vi "Power Output Append Group Data Fields.vi"(10 "Power Output Results":T1={"Measurement Cycles"=0, "Measurement Data"=[], "Pass?"=FALSE, "Instruments to Use"={"PIM Instrument Record"={"ixInstrument"=0, "sxInstrumentId"="", "sDriverId"="", "sDriverType"="", "sSerialNumber"="", "tLastCalibration"=timestamp(0 s since 1904-01-01), "tCalibrationDue"=timestamp(0 s since 1904-01-01), "sConfiguration"=""}, "PWM Instrument Record"={"ixInstrument"=0, "sxInstrumentId"="", "sDriverId"="", "sDriverType"="", "sSerialNumber"="", "tLastCalibration"=timestamp(0 s since 1904-01-01), "tCalibrationDue"=timestamp(0 s since 1904-01-01), "sConfiguration"=""}}, "Power Output Test Parameters"={"Stimulus"={"Frequency Type"=enum."Band Edges", "Frequency Ranges"=[], "TX 1 Frequency (MHz)"={"Min"=0.0, "Max"=0.0}, "TX 2 Frequency (MHz)"={"Min"=0.0, "Max"=0.0}, "RX Frequency (MHz)"={"Min"=0.0, "Max"=0.0}, "Pad Model Number"="", "Pad Serial Number"="", "Pad Values"=[]}, "Measurement"={"DUT Port"=enum."Port 1", "Direction"=0, "Frequency Step Size"=0}, "Display"={"Frequency"={"Min"=-1.0, "Max"=-1.0}, "Power"={"Min"=-1, "Max"=-1}}, "Limit"={"Min Power (dBm)"=44.0}, "Calibration"={"Calibrated?"=FALSE}}, "Calculated Values"={"C1 PWM Power Min (dBm)"=0.0, "C1 PWM Power Max (dBm)"=0.0, "C1 PIM Power Min (dBm)"=0.0, "C1 PIM Power Max (dBm)"=0.0, "C2 PWM Power Min (dBm)"=0.0, "C2 PWM Power Max (dBm)"=0.0, "C2 PIM Power Min (dBm)"=0.0, "C2 PIM Power Max (dBm)"=0.0}} {"Power Output Test Parameters"."Measurement"."Frequency Step Size" items=["0.2", "0.4", "1.0", "2.0", "4.0"]; "Power Output Test Parameters"."Measurement"."Direction" items=["Reverse", "Forward", "Auxiliary"]}, 11 "Fields In":T14[](array[typedef])) -> (3 "Fields Out":T14[](array[typedef]))   [LabVIEW 2011]
uses:
  server/database/Fields/Field Record.ctl
  server/database/Fields/Field DataTypes.ctl
  server/database/Fields/Field NextItem.ctl
  TypeDefs/Power Output Results.ctl
  TypeDefs/Power Output Measurement Data.ctl
  server/database/Stations/Instruments/Instrument Record.ctl
  TypeDefs/Power Output Test Parameters.ctl
  TypeDefs/Power Output Stimulus Parameters.ctl
  TypeDefs/Power Output Measurement Parameters.ctl
  SI.LIB/PIM.LIB/HW IO/DUTport.ctl
  SI.LIB/PIM.LIB/HW IO/MeasMode.ctl
  SI.LIB/PIM.LIB/HW IO/PIM Sweep Step Size.ctl
  TypeDefs/Power Output Display Parameters.ctl
  TypeDefs/Power Output Limit Parameters.ctl
  TypeDefs/Power Output Calibration State.ctl
  TypeDefs/Power Output Calculated Values.ctl
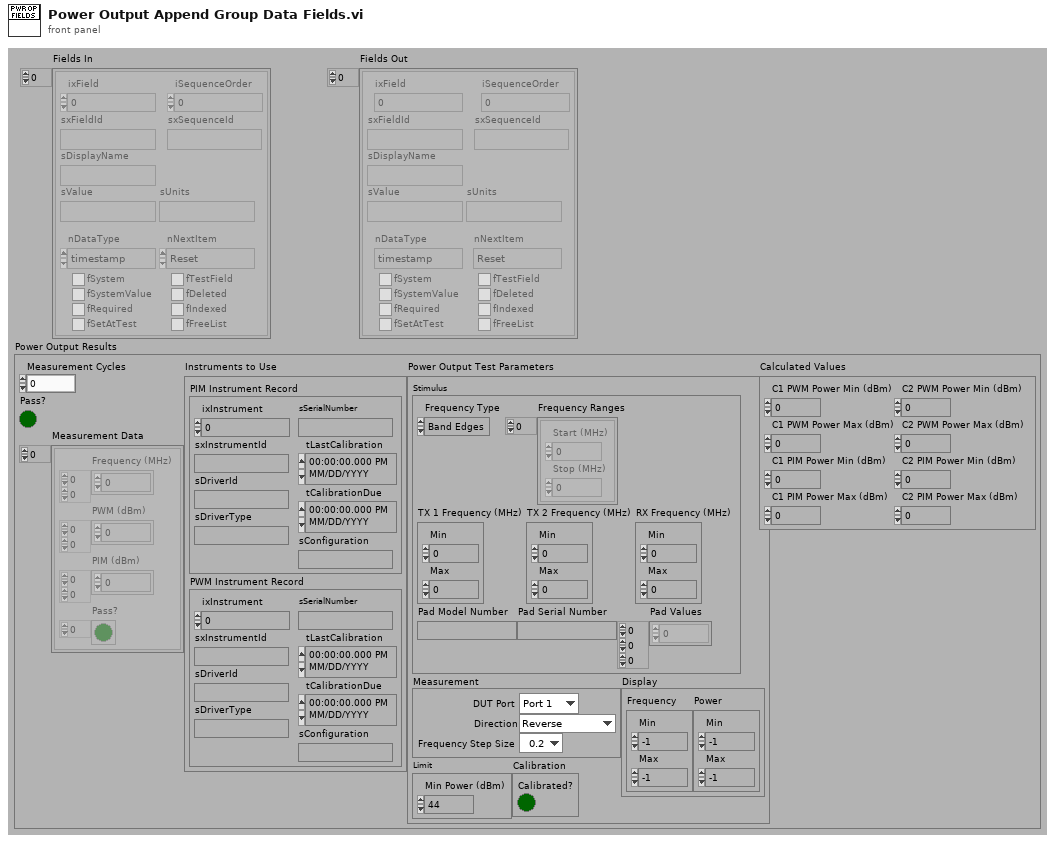
[diagram p1: front panel]
types:
  T1 = typedef "Power Output Results.ctl" = cluster{"Measurement Cycles":i32, "Measurement Data":T2[], "Pass?":bool, "Instruments to Use":cluster{"PIM Instrument Record":T3, "PWM Instrument Record":T3}, "Power Output Test Parameters":T4, "Calculated Values":T13}
  T2 = typedef "Power Output Measurement Data.ctl" = cluster{"Frequency (MHz)":dbl[][], "PWM (dBm)":dbl[][], "PIM (dBm)":dbl[][], "Pass?":bool[]}
  T3 = typedef "Instrument Record.ctl" = cluster{"ixInstrument":i32, "sxInstrumentId":string, "sDriverId":string, "sDriverType":string, "sSerialNumber":string, "tLastCalibration":timestamp, "tCalibrationDue":timestamp, "sConfiguration":string}
  T4 = typedef "Power Output Test Parameters.ctl" = cluster{"Stimulus":T5, "Measurement":T6, "Display":T10, "Limit":T11, "Calibration":T12}
  T5 = typedef "Power Output Stimulus Parameters.ctl" = cluster{"Frequency Type":enum16{"Band Edges", "Custom"}, "Frequency Ranges":cluster{"Start (MHz)":dbl, "Stop (MHz)":dbl}[], "TX 1 Frequency (MHz)":cluster{"Min":dbl, "Max":dbl}, "TX 2 Frequency (MHz)":cluster{"Min":dbl, "Max":dbl}, "RX Frequency (MHz)":cluster{"Min":dbl, "Max":dbl}, "Pad Model Number":string, "Pad Serial Number":string, "Pad Values":dbl[][][]}
  T6 = typedef "Power Output Measurement Parameters.ctl" = cluster{"DUT Port":T7, "Direction":T8, "Frequency Step Size":T9}
  T7 = typedef "DUTport.ctl" = enum16{"Port 1", "Port 2"}
  T8 = typedef "MeasMode.ctl" = u16
  T9 = typedef "PIM Sweep Step Size.ctl" = u16
  T10 = typedef "Power Output Display Parameters.ctl" = cluster{"Frequency":cluster{"Min":dbl, "Max":dbl}, "Power":cluster{"Min":i32, "Max":i32}}
  T11 = typedef "Power Output Limit Parameters.ctl" = cluster{"Min Power (dBm)":dbl}
  T12 = typedef "Power Output Calibration State.ctl" = cluster{"Calibrated?":bool}
  T13 = typedef "Power Output Calculated Values.ctl" = cluster{"C1 PWM Power Min (dBm)":dbl, "C1 PWM Power Max (dBm)":dbl, "C1 PIM Power Min (dBm)":dbl, "C1 PIM Power Max (dBm)":dbl, "C2 PWM Power Min (dBm)":dbl, "C2 PWM Power Max (dBm)":dbl, "C2 PIM Power Min (dBm)":dbl, "C2 PIM Power Max (dBm)":dbl}
  T14 = typedef "Field Record.ctl" = cluster{"ixField":i32, "iSequenceOrder":i32, "sxFieldId":string, "sxSequenceId":string, "sDisplayName":string, "sValue":string, "sUnits":string, "nDataType":T15, "nNextItem":T16, "fSystem":bool, "fSystemValue":bool, "fRequired":bool, "fSetAtTest":bool, "fTestField":bool, "fDeleted":bool, "fIndexed":bool, "fFreeList":bool}
  T15 = typedef "Field DataTypes.ctl" = enum32{"text", "numeric", "list", "timestamp", "boolean"}
  T16 = typedef "Field NextItem.ctl" = enum32{"Reset", "Retain", "Auto-Increment"}
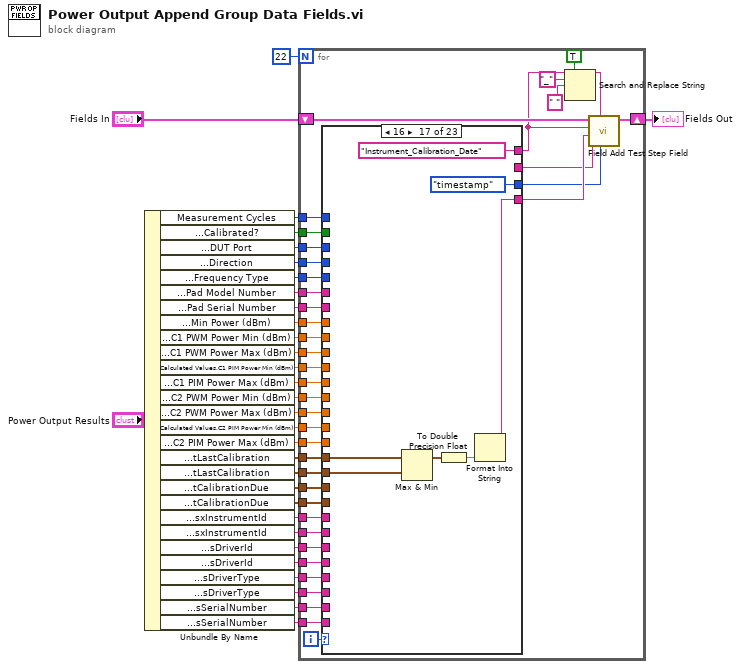
[diagram p0: block diagram]
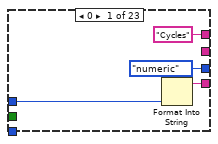
[diagram p2: hidden frame]
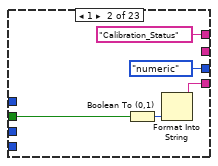
[diagram p3: hidden frame]
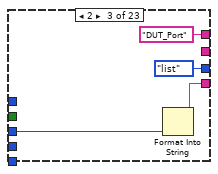
[diagram p4: hidden frame]
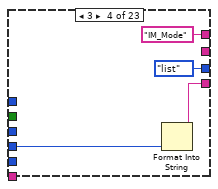
[diagram p5: hidden frame]
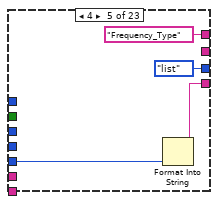
[diagram p6: hidden frame]
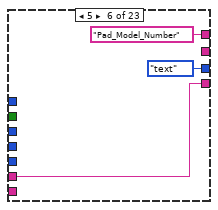
[diagram p7: hidden frame]
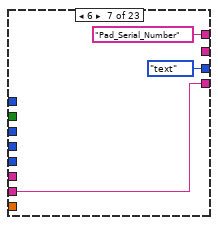
[diagram p8: hidden frame]
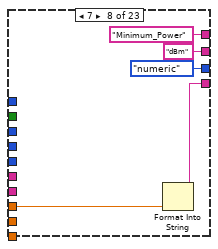
[diagram p9: hidden frame]
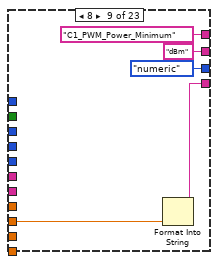
[diagram p10: hidden frame]
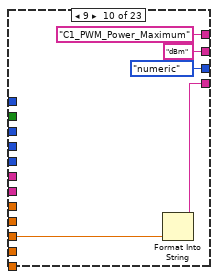
[diagram p11: hidden frame]
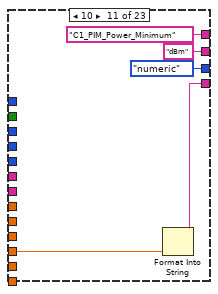
[diagram p12: hidden frame]
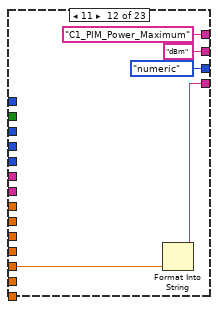
[diagram p13: hidden frame]
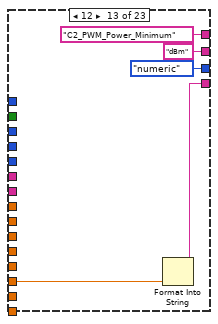
[diagram p14: hidden frame]
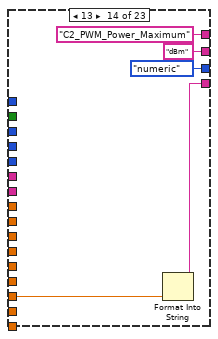
[diagram p15: hidden frame]
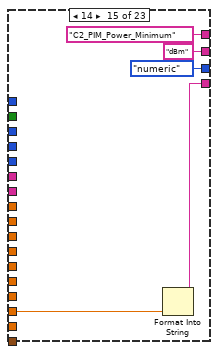
[diagram p16: hidden frame]
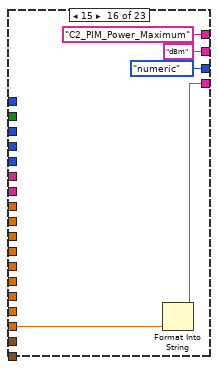
[diagram p17: hidden frame]
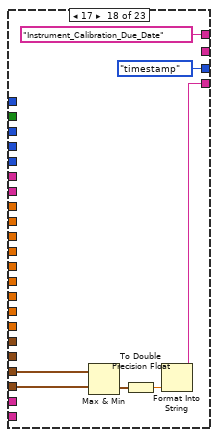
[diagram p18: hidden frame]
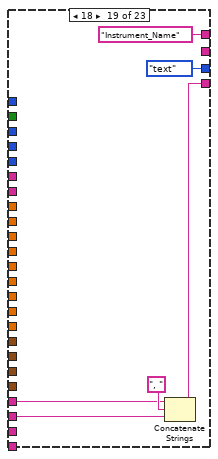
[diagram p19: hidden frame]
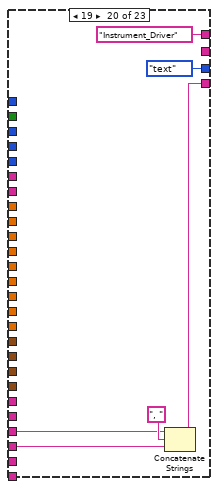
[diagram p20: hidden frame]
diagram:
  n1 = Unbundle By Name("Power Output Results") -> ("Measurement Cycles"=w28:i32, "Power Output Test Parameters.Calibration.Calibrated?"=w27:bool, "Power Output Test Parameters.Measurement.DUT Port"=w26:T7, "Power Output Test Parameters.Measurement.Direction"=w18:T8, "Power Output Test Parameters.Stimulus.Frequency Type"=w19:enum16{"Band Edges", "Custom"}, "Power Output Test Parameters.Stimulus.Pad Model Number"=w11:string, "Power Output Test Parameters.Stimulus.Pad Serial Number"=w10:string, "Power Output Test Parameters.Limit.Min Power (dBm)"=w9:dbl, "Calculated Values.C1 PWM Power Min (dBm)"=w8:dbl, "Calculated Values.C1 PWM Power Max (dBm)"=w7:dbl, "Calculated Values.C1 PIM Power Min (dBm)"=w6:dbl, "Calculated Values.C1 PIM Power Max (dBm)"=w5:dbl, "Calculated Values.C2 PWM Power Min (dBm)"=w4:dbl, "Calculated Values.C2 PWM Power Max (dBm)"=w3:dbl, "Calculated Values.C2 PIM Power Min (dBm)"=w2:dbl, "Calculated Values.C2 PIM Power Max (dBm)"=w1:dbl, "Instruments to Use.PIM Instrument Record.tLastCalibration"=w25:timestamp, "Instruments to Use.PWM Instrument Record.tLastCalibration"=w12:timestamp, "Instruments to Use.PIM Instrument Record.tCalibrationDue"=w24:timestamp, "Instruments to Use.PWM Instrument Record.tCalibrationDue"=w13:timestamp, "Instruments to Use.PIM Instrument Record.sxInstrumentId"=w23:string, "Instruments to Use.PWM Instrument Record.sxInstrumentId"=w17:string, "Instruments to Use.PIM Instrument Record.sDriverId"=w22:string, "Instruments to Use.PWM Instrument Record.sDriverId"=w16:string, "Instruments to Use.PIM Instrument Record.sDriverType"=w21:string, "Instruments to Use.PWM Instrument Record.sDriverType"=w15:string, "Instruments to Use.PIM Instrument Record.sSerialNumber"=w20:string, "Instruments to Use.PWM Instrument Record.sSerialNumber"=w14:string)
  n2 = for {
    N: 22 -> [_]
    shift-right: [w69] -> w31
    shift-left: "Fields In" -> [w70]
    tunnel: w28 -> [w65]
    tunnel: w27 -> [w64]
    tunnel: w26 -> [w63]
    tunnel: w25 -> [w62]
    tunnel: w24 -> [w61]
    tunnel: w23 -> [w60]
    tunnel: w22 -> [w59]
    tunnel: w21 -> [w58]
    tunnel: w20 -> [w57]
    tunnel: w19 -> [w56]
    tunnel: w18 -> [w50]
    tunnel: w17 -> [w49]
    tunnel: w16 -> [w48]
    tunnel: w15 -> [w47]
    tunnel: w14 -> [w46]
    tunnel: w13 -> [w45]
    tunnel: w12 -> [w44]
    tunnel: w11 -> [w43]
    tunnel: w10 -> [w42]
    tunnel: w9 -> [w41]
    tunnel: w8 -> [w40]
    tunnel: w7 -> [w39]
    tunnel: w6 -> [w38]
    tunnel: w5 -> [w37]
    tunnel: w4 -> [w36]
    tunnel: w3 -> [w35]
    tunnel: w2 -> [w34]
    tunnel: w1 -> [w33]
    i -> [w71]
    n3 = case shown="16" w71 {
      tunnel: ["Cycles" ("Field_ID") "Calibration_Status" ("Field_ID") "DUT_Port" ("Field_ID") "IM_Mode" ("Field_ID") "Frequency_Type" ("Field_ID") "Pad_Model_Number" ("Field_ID") "Pad_Serial_Number" ("Field_ID") "Minimum_Power" ("Field_ID") "C1_PWM_Power_Minimum" ("Field_ID") "C1_PWM_Power_Maximum" ("Field_ID") "C1_PIM_Power_Minimum" ("Field_ID") "C1_PIM_Power_Maximum" ("Field_ID") "C2_PWM_Power_Minimum" ("Field_ID") "C2_PWM_Power_Maximum" ("Field_ID") "C2_PIM_Power_Minimum" ("Field_ID") "C2_PIM_Power_Maximum" ("Field_ID") "Instrument_Calibration_Date" ("Field_ID") "Instrument_Calibration_Due_Date" ("Field_ID") "Instrument_Name" ("Field_ID") "Instrument_Driver" ("Field_ID") "Instrument_Type" ("Field_ID") "Instrument_Serial_Number" ("Field_ID") _] -> w52
      tunnel: [Field_DataTypes."numeric" ("Data Type") Field_DataTypes."numeric" ("Data Type") Field_DataTypes."list" ("Data Type") Field_DataTypes."list" ("Data Type") Field_DataTypes."list" ("Data Type") Field_DataTypes."text" ("Data Type") Field_DataTypes."text" ("Data Type") Field_DataTypes."numeric" ("Data Type") Field_DataTypes."numeric" ("Data Type") Field_DataTypes."numeric" ("Data Type") Field_DataTypes."numeric" ("Data Type") Field_DataTypes."numeric" ("Data Type") Field_DataTypes."numeric" ("Data Type") Field_DataTypes."numeric" ("Data Type") Field_DataTypes."numeric" ("Data Type") Field_DataTypes."numeric" ("Data Type") Field_DataTypes."timestamp" ("Data Type") Field_DataTypes."timestamp" ("Data Type") Field_DataTypes."text" ("Data Type") Field_DataTypes."text" ("Data Type") Field_DataTypes."text" ("Data Type") Field_DataTypes."text" ("Data Type") Field_DataTypes."text" ("Data Type")] -> w67
      tunnel: [w74 w79 w83 w87 w90 w93 w96 w101 w106 w111 w116 w121 w126 w131 w136 w141 w146 w151 w159 w164 w171 w177 _] -> w68
      tunnel: [_ _ _ _ _ _ _ "dBm" "dBm" "dBm" "dBm" "dBm" "dBm" "dBm" "dBm" "dBm" _ _ _ _ _ _ ""] -> w66
      tunnel: w65 -> [w72 _ _ _ _ _ _ _ _ _ _ _ _ _ _ _ _ _ _ _ _ _ _]
      tunnel: w64 -> [_ w77 _ _ _ _ _ _ _ _ _ _ _ _ _ _ _ _ _ _ _ _ _]
      tunnel: w63 -> [_ _ w81 _ _ _ _ _ _ _ _ _ _ _ _ _ _ _ _ _ _ _ _]
      tunnel: w62 -> [_ _ _ _ _ _ _ _ _ _ _ _ _ _ _ _ w145 _ _ _ _ _ _]
      tunnel: w61 -> [_ _ _ _ _ _ _ _ _ _ _ _ _ _ _ _ _ w153 _ _ _ _ _]
      tunnel: w60 -> [_ _ _ _ _ _ _ _ _ _ _ _ _ _ _ _ _ _ w160 _ _ _ _]
      tunnel: w59 -> [_ _ _ _ _ _ _ _ _ _ _ _ _ _ _ _ _ _ _ w166 _ _ _]
      tunnel: w58 -> [_ _ _ _ _ _ _ _ _ _ _ _ _ _ _ _ _ _ _ _ w172 _ _]
      tunnel: w57 -> [_ _ _ _ _ _ _ _ _ _ _ _ _ _ _ _ _ _ _ _ _ w178 _]
      tunnel: w56 -> [_ _ _ _ w89 _ _ _ _ _ _ _ _ _ _ _ _ _ _ _ _ _ _]
      tunnel: w50 -> [_ _ _ w85 _ _ _ _ _ _ _ _ _ _ _ _ _ _ _ _ _ _ _]
      tunnel: w49 -> [_ _ _ _ _ _ _ _ _ _ _ _ _ _ _ _ _ _ w158 _ _ _ _]
      tunnel: w48 -> [_ _ _ _ _ _ _ _ _ _ _ _ _ _ _ _ _ _ _ w165 _ _ _]
      tunnel: w47 -> [_ _ _ _ _ _ _ _ _ _ _ _ _ _ _ _ _ _ _ _ w170 _ _]
      tunnel: w46 -> [_ _ _ _ _ _ _ _ _ _ _ _ _ _ _ _ _ _ _ _ _ w176 _]
      tunnel: w45 -> [_ _ _ _ _ _ _ _ _ _ _ _ _ _ _ _ _ w152 _ _ _ _ _]
      tunnel: w44 -> [_ _ _ _ _ _ _ _ _ _ _ _ _ _ _ _ w144 _ _ _ _ _ _]
      tunnel: w43 -> [_ _ _ _ _ w93 _ _ _ _ _ _ _ _ _ _ _ _ _ _ _ _ _]
      tunnel: w42 -> [_ _ _ _ _ _ w96 _ _ _ _ _ _ _ _ _ _ _ _ _ _ _ _]
      tunnel: w41 -> [_ _ _ _ _ _ _ w100 _ _ _ _ _ _ _ _ _ _ _ _ _ _ _]
      tunnel: w40 -> [_ _ _ _ _ _ _ _ w104 _ _ _ _ _ _ _ _ _ _ _ _ _ _]
      tunnel: w39 -> [_ _ _ _ _ _ _ _ _ w109 _ _ _ _ _ _ _ _ _ _ _ _ _]
      tunnel: w38 -> [_ _ _ _ _ _ _ _ _ _ w114 _ _ _ _ _ _ _ _ _ _ _ _]
      tunnel: w37 -> [_ _ _ _ _ _ _ _ _ _ _ w119 _ _ _ _ _ _ _ _ _ _ _]
      tunnel: w36 -> [_ _ _ _ _ _ _ _ _ _ _ _ w124 _ _ _ _ _ _ _ _ _ _]
      tunnel: w35 -> [_ _ _ _ _ _ _ _ _ _ _ _ _ w129 _ _ _ _ _ _ _ _ _]
      tunnel: w34 -> [_ _ _ _ _ _ _ _ _ _ _ _ _ _ w134 _ _ _ _ _ _ _ _]
      tunnel: w33 -> [_ _ _ _ _ _ _ _ _ _ _ _ _ _ _ w139 _ _ _ _ _ _ _]
      frame 0 {
        n4 = Format Into String(w72) -> (resulting string=w74:string)  [unwired: 3 in, 1 out]
      }
      frame 1 {
        n5 = Boolean To (0,1)(Boolean=w77) -> (0, 1=w76:i16)
        n6 = Format Into String(w76) -> (resulting string=w79:string)  [unwired: 3 in, 1 out]
      }
      frame 2 {
        n7 = Format Into String(w81) -> (resulting string=w83:string)  [unwired: 3 in, 1 out]
      }
      frame 3 {
        n8 = Format Into String(w85) -> (resulting string=w87:string)  [unwired: 3 in, 1 out]
      }
      frame 4 {
        n9 = Format Into String(w89) -> (resulting string=w90:string)  [unwired: 3 in, 1 out]
      }
      frame 5 {
      }
      frame 6 {
      }
      frame 7 {
        n10 = Format Into String(w100) -> (resulting string=w101:string)  [unwired: 3 in, 1 out]
      }
      frame 8 {
        n11 = Format Into String(w104) -> (resulting string=w106:string)  [unwired: 3 in, 1 out]
      }
      frame 9 {
        n12 = Format Into String(w109) -> (resulting string=w111:string)  [unwired: 3 in, 1 out]
      }
      frame 10 {
        n13 = Format Into String(w114) -> (resulting string=w116:string)  [unwired: 3 in, 1 out]
      }
      frame 11 {
        n14 = Format Into String(w119) -> (resulting string=w121:string)  [unwired: 3 in, 1 out]
      }
      frame 12 {
        n15 = Format Into String(w124) -> (resulting string=w126:string)  [unwired: 3 in, 1 out]
      }
      frame 13 {
        n16 = Format Into String(w129) -> (resulting string=w131:string)  [unwired: 3 in, 1 out]
      }
      frame 14 {
        n17 = Format Into String(w134) -> (resulting string=w136:string)  [unwired: 3 in, 1 out]
      }
      frame 15 {
        n18 = Format Into String(w139) -> (resulting string=w141:string)  [unwired: 3 in, 1 out]
      }
      frame 16 {
        n19 = Max & Min(x=w145, y=w144) -> (max(x,y)=w147:timestamp)  [unwired: 1 out]
        n20 = To Double Precision Float(number=w147) -> (double precision float=w148:dbl)
        n21 = Format Into String(w148) -> (resulting string=w146:string)  [unwired: 3 in, 1 out]
      }
      frame 17 {
        n22 = Max & Min(x=w153, y=w152) -> (min(x,y)=w154:timestamp)  [unwired: 1 out]
        n23 = To Double Precision Float(number=w154) -> (double precision float=w155:dbl)
        n24 = Format Into String(w155) -> (resulting string=w151:string)  [unwired: 3 in, 1 out]
      }
      frame 18 {
        n25 = Concatenate Strings(w160, ", ", w158) -> (w159:string)
      }
      frame 19 {
        n26 = Concatenate Strings(w166, ", ", w165) -> (w164:string)
      }
      frame 20 {
        n27 = Concatenate Strings(w172, ", ", w170) -> (w171:string)
      }
      frame 21 {
        n28 = Concatenate Strings(w178, ", ", w176) -> (w177:string)
      }
      frame Default {
      }
    }
    n29 = Search and Replace String(replace all?=TRUE ("replace all? (F)"), input string=w52, search string="_", replace string=" " ("replace string (\"\")")) -> (result string=w51:string)  [unwired: 1 in, 6 out]
    n30 = call "Field Add Test Step Field.vi"("nDataType"=w67, "sDisplayName"=w51, "sUnits"=w66, "sValue"=w68, "sxFieldId"=w52, "Fields In"=w70) -> ("Fields Out"=w69:T14[])  [unwired: 5 out]
  }
  "Fields Out" <- w31
